vi "Configuration To Tree.vi"(4 "TargetIndex":u16, 6 "ProjectPath":path, 7 "Owning Tree":string, 8 "error in":errorcluster, 9 "Mode":T2, 11 "Tree Manager in":T1) -> (0 "error out":errorcluster, 3 "Tree Manager out":T1)   [LabVIEW 2020]
uses:
  <vilib>/addons/analyzer/_analyzerctrls.llb/VIAnCtl AnalyzeMode.ctl
  <vilib>/addons/analyzer/VIAnCFGDataStructure/Tree Manager/Typedefs/Session Handle.ctl
  <vilib>/addons/analyzer/VIAnCFGDataStructure/Tree Manager/Tree.lvclass
  <vilib>/addons/analyzer/VIAnCFGDataStructure/Data Types/Int/Int.lvclass/Int.ctl
  <vilib>/addons/analyzer/VIAnCFGDataStructure/Data Types/Bool/Bool.lvclass/Bool.ctl
  <vilib>/addons/analyzer/VIAnCFGDataStructure/Data Types/Path/Path.lvclass/Path.ctl
  <vilib>/addons/analyzer/VIAnCFGDataStructure/Data Types/Bool/To Bool Tree Data.vi
  <vilib>/addons/analyzer/VIAnCFGDataStructure/Data Types/Path/To Path Tree Data.vi
  <vilib>/addons/analyzer/VIAnCFGDataStructure/Data Types/Int/To Integer Tree Data.vi
  <vilib>/addons/analyzer/VIAnCFGDataStructure/Data Types/Bool/Bool.lvclass
  e:/builds/penguin/labview/branches/2020/dev/dist/vi.lib/addons/analyzer/VIAnCFGDataStructure/Tree Data/Tree Data.lvclass
  <vilib>/addons/analyzer/VIAnCFGDataStructure/Data Types/Path/Path.lvclass
  <vilib>/addons/analyzer/VIAnCFGDataStructure/Data Types/Int/Int.lvclass
  <vilib>/addons/analyzer/_vianuishared.llb/VIAnUI CFG File Info Global.vi
  <vilib>/addons/analyzer/VIAnCFGDataStructure/Tree Manager/API/Set Attribute Tree Data.vi
  e:/builds/penguin/labview/branches/2020/dev/dist/vi.lib/addons/analyzer/VIAnCFGDataStructure/Data Types/Bool/Bool.lvclass
  e:/builds/penguin/labview/branches/2020/dev/dist/vi.lib/addons/analyzer/VIAnCFGDataStructure/Data Types/Path/Path.lvclass
  e:/builds/penguin/labview/branches/2020/dev/dist/vi.lib/addons/analyzer/VIAnCFGDataStructure/Data Types/Int/Int.lvclass
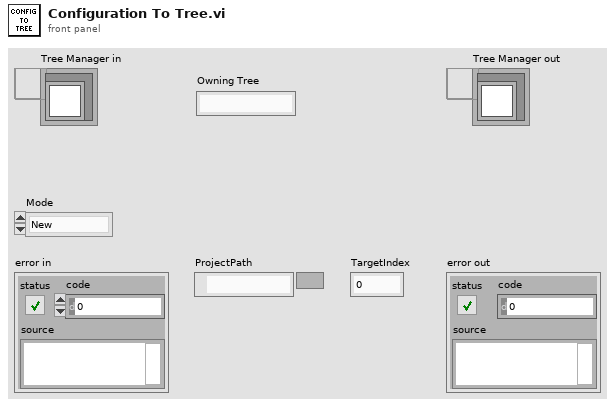
[diagram p1: front panel]
types:
  T1 = typedef "NI_VIAnCFGDataStructure.lvlib/Tree.lvclass/Session Handle.ctl" = refnum<data-value>
  T2 = typedef "VIAnCtl AnalyzeMode.ctl" = enum16{"New", "Load", "AnalyzeThis", "AnalyzeProj"}
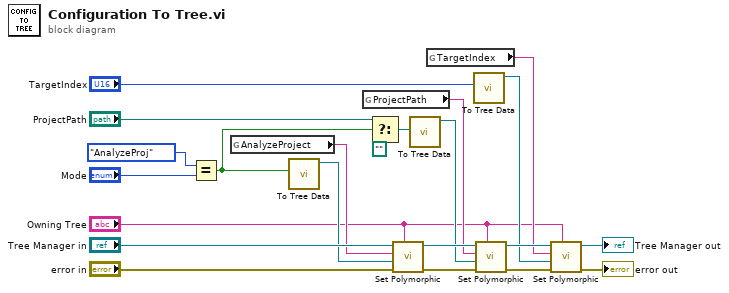
[diagram p0: block diagram]
diagram:
  n1 = Equal?(x=VIAnCtl_AnalyzeMode."AnalyzeProj", y="Mode") -> (x = y?=w4:bool)
  n2 = global read "VIAnUI CFG File Info Global.vi" "AnalyzeProject"() -> (w8:string)
  n3 = call-poly <vilib>:"To Tree Data.vi"("Boolean"=w4) -> ("Bool Tree Data"=w14:refnum<class "Bool.lvclass">)  [unwired: 10 in]
  n4 = global read "VIAnUI CFG File Info Global.vi" "ProjectPath"() -> (w9:string)
  n5 = Select(t="ProjectPath", s=w4, f=path "") -> (s? t:f=w3:path)
  n6 = call-poly <vilib>:"Set Polymorphic.vi"("Tree ID"="Owning Tree", "Error In"="error in", "Attribute Value"=w14, "Attribute Name"=w8, "Tree Manager"="Tree Manager in") -> ("Error Out"=w19:errorcluster, "Tree Manager"=w18:T1)  [unwired: 4 in, 1 out]
  n7 = call-poly <vilib>:"To Tree Data.vi"("Path"=w3) -> ("Path Tree Data"=w13:refnum<class "Path.lvclass">)  [unwired: 10 in]
  n8 = global read "VIAnUI CFG File Info Global.vi" "TargetIndex"() -> (w10:string)
  n9 = call-poly <vilib>:"To Tree Data.vi"("Integer"="TargetIndex") -> ("Integer Tree Data"=w12:refnum<class "Int.lvclass">)  [unwired: 10 in]
  n10 = call-poly <vilib>:"Set Polymorphic.vi"("Tree ID"="Owning Tree", "Error In"=w19, "Attribute Value"=w13, "Attribute Name"=w9, "Tree Manager"=w18) -> ("Error Out"=w21:errorcluster, "Tree Manager"=w20:T1)  [unwired: 4 in, 1 out]
  n11 = call-poly <vilib>:"Set Polymorphic.vi"("Tree ID"="Owning Tree", "Error In"=w21, "Attribute Value"=w12, "Attribute Name"=w10, "Tree Manager"=w20) -> ("Error Out"=→"error out":errorcluster, "Tree Manager"=→"Tree Manager out":T1)  [unwired: 4 in, 1 out]
